vi "BooleanGame.vi"() -> ()   [LabVIEW 2015]
panel:
  out "String":string
  in  "Select a Puzzle":u16(ring) items=["None", "Puzzle 1", "Puzzle 2", "Puzzle 3", "Puzzle 4", "Puzzle 5", "Impossible Challenge"]
  in  "reset":bool
  in  "stop":bool
  in  "33":bool
  in  "23":bool
  in  "13":bool
  in  "32":bool
  in  "22":bool
  in  "12":bool
  in  "31":bool
  in  "21":bool
  in  "11":bool
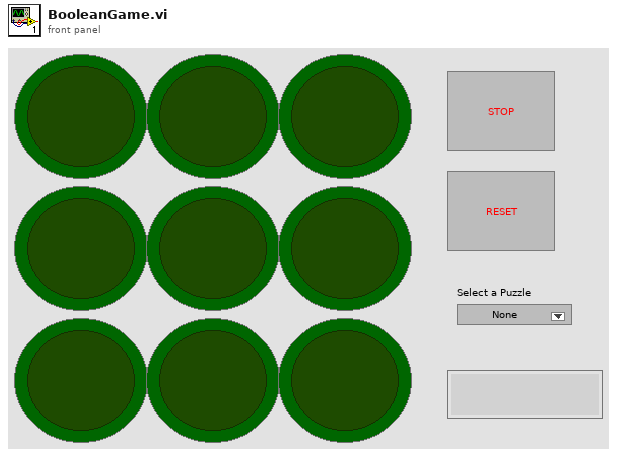
[diagram p1: front panel]
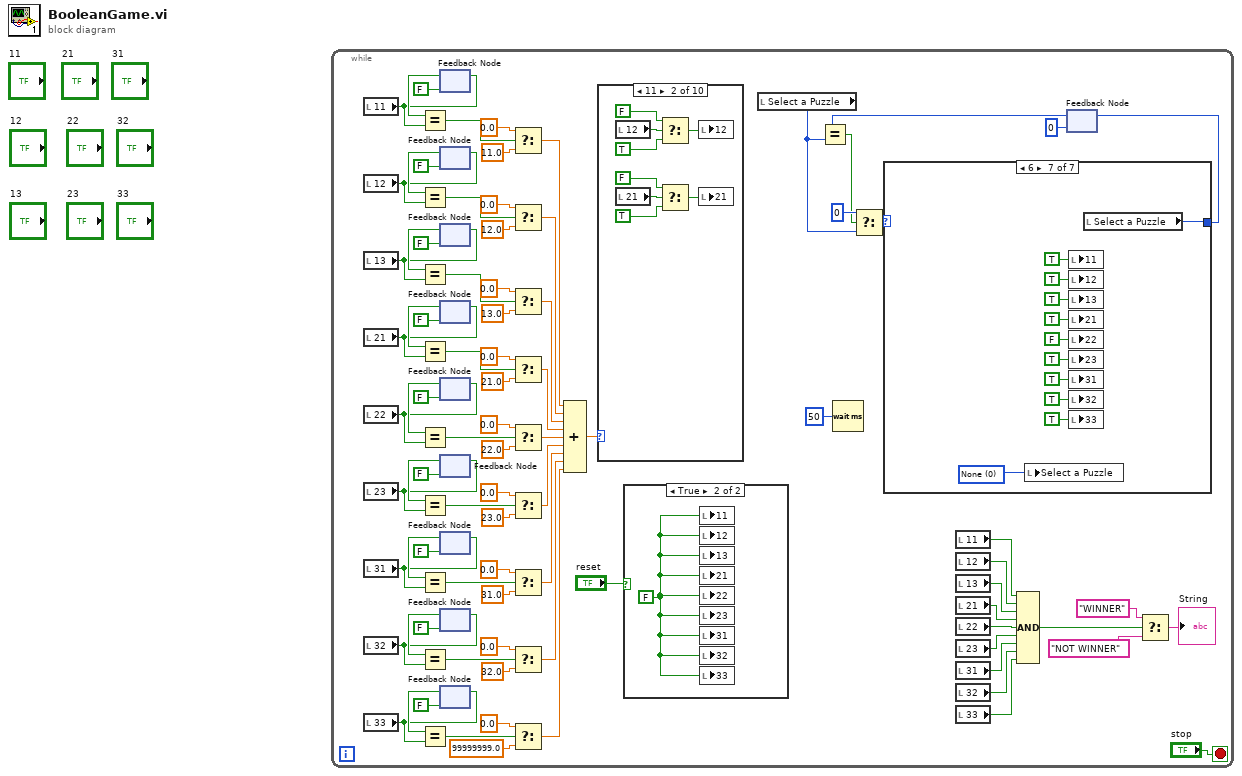
[diagram p0: block diagram]
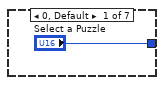
[diagram p2: hidden frame]
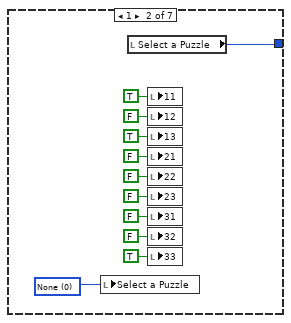
[diagram p3: hidden frame]
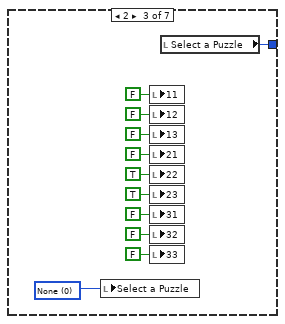
[diagram p4: hidden frame]
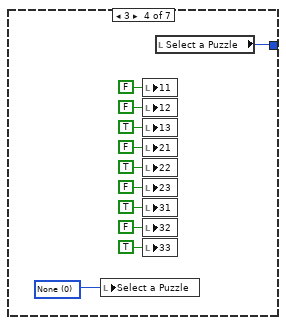
[diagram p5: hidden frame]
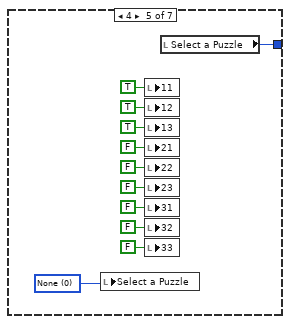
[diagram p6: hidden frame]
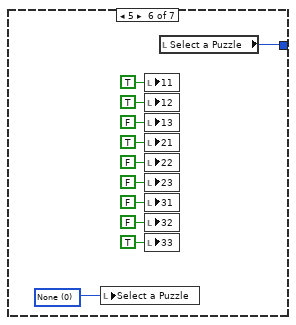
[diagram p7: hidden frame]
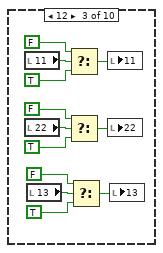
[diagram p10: hidden frame]
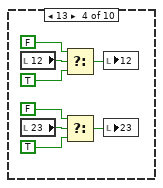
[diagram p11: hidden frame]
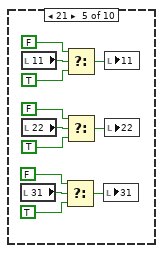
[diagram p12: hidden frame]
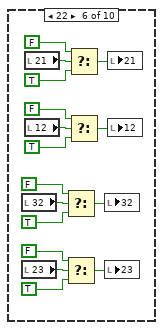
[diagram p13: hidden frame]
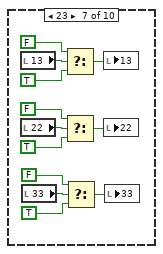
[diagram p14: hidden frame]
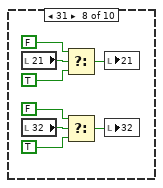
[diagram p15: hidden frame]
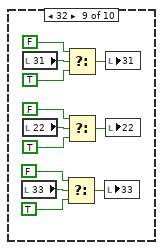
[diagram p16: hidden frame]
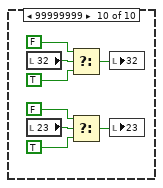
[diagram p17: hidden frame]
diagram:
  n1 = while {
    stop <- "stop" stop-if-true
    n2 = local read "11"() -> (w31:bool)
    n3 = local read "12"() -> (w30:bool)
    n4 = local read "13"() -> (w29:bool)
    n5 = local read "21"() -> (w28:bool)
    n6 = local read "22"() -> (w27:bool)
    n7 = local read "23"() -> (w26:bool)
    n8 = local read "31"() -> (w25:bool)
    n9 = local read "32"() -> (w24:bool)
    n10 = local read "33"() -> (w23:bool)
    n11 = feedback #1(FALSE) -> (w57:bool)
    n12 = Equal?(x=w57, y=w31) -> (x = y?=w58:bool)
    n13 = feedback-in #1(w31) -> ()
    n14 = feedback #2(FALSE) -> (w55:bool)
    n15 = Equal?(x=w55, y=w30) -> (x = y?=w56:bool)
    n16 = feedback-in #2(w30) -> ()
    n17 = feedback #3(FALSE) -> (w53:bool)
    n18 = Equal?(x=w53, y=w29) -> (x = y?=w54:bool)
    n19 = feedback-in #3(w29) -> ()
    n20 = feedback #4(FALSE) -> (w51:bool)
    n21 = Equal?(x=w51, y=w28) -> (x = y?=w52:bool)
    n22 = feedback-in #4(w28) -> ()
    n23 = feedback #5(FALSE) -> (w49:bool)
    n24 = Equal?(x=w49, y=w27) -> (x = y?=w50:bool)
    n25 = feedback-in #5(w27) -> ()
    n26 = feedback #6(FALSE) -> (w47:bool)
    n27 = Equal?(x=w47, y=w26) -> (x = y?=w48:bool)
    n28 = feedback-in #6(w26) -> ()
    n29 = feedback #7(FALSE) -> (w45:bool)
    n30 = Equal?(x=w45, y=w25) -> (x = y?=w46:bool)
    n31 = feedback-in #7(w25) -> ()
    n32 = feedback #8(FALSE) -> (w43:bool)
    n33 = Equal?(x=w43, y=w24) -> (x = y?=w44:bool)
    n34 = feedback-in #8(w24) -> ()
    n35 = feedback #9(FALSE) -> (w41:bool)
    n36 = Equal?(x=w41, y=w23) -> (x = y?=w42:bool)
    n37 = feedback-in #9(w23) -> ()
    n38 = Select(t=0.0, s=w58, f=11.0) -> (s? t:f=w68:dbl)
    n39 = Select(t=0.0, s=w56, f=12.0) -> (s? t:f=w67:dbl)
    n40 = Select(t=0.0, s=w54, f=13.0) -> (s? t:f=w66:dbl)
    n41 = Select(t=0.0, s=w52, f=21.0) -> (s? t:f=w65:dbl)
    n42 = Select(t=0.0, s=w50, f=22.0) -> (s? t:f=w64:dbl)
    n43 = Select(t=0.0, s=w48, f=23.0) -> (s? t:f=w63:dbl)
    n44 = Select(t=0.0, s=w46, f=31.0) -> (s? t:f=w62:dbl)
    n45 = Select(t=0.0, s=w44, f=32.0) -> (s? t:f=w61:dbl)
    n46 = Select(t=0.0, s=w42, f=99999999.0) -> (s? t:f=w60:dbl)
    n47 = Compound Arithmetic op=ADD(w68, w67, w66, w65, w64, w63, w62, w61, w60) -> (w59:dbl)
    n48 = case shown="11" w59 {
      frame 0, Default {
      }
      frame 11 {
        n49 = local read "12"() -> (w156:bool)
        n50 = local read "21"() -> (w163:bool)
        n51 = Select(t=FALSE, s=w156, f=TRUE) -> (s? t:f=w159:bool)
        n52 = Select(t=FALSE, s=w163, f=TRUE) -> (s? t:f=w160:bool)
        n53 = local write "12"(w159) -> ()
        n54 = local write "21"(w160) -> ()
      }
      frame 12 {
        n55 = local read "11"() -> (w168:bool)
        n56 = local read "22"() -> (w175:bool)
        n57 = local read "13"() -> (w164:bool)
        n58 = Select(t=FALSE, s=w168, f=TRUE) -> (s? t:f=w171:bool)
        n59 = Select(t=FALSE, s=w175, f=TRUE) -> (s? t:f=w172:bool)
        n60 = Select(t=FALSE, s=w164, f=TRUE) -> (s? t:f=w167:bool)
        n61 = local write "11"(w171) -> ()
        n62 = local write "22"(w172) -> ()
        n63 = local write "13"(w167) -> ()
      }
      frame 13 {
        n64 = local read "12"() -> (w176:bool)
        n65 = local read "23"() -> (w183:bool)
        n66 = Select(t=FALSE, s=w176, f=TRUE) -> (s? t:f=w179:bool)
        n67 = Select(t=FALSE, s=w183, f=TRUE) -> (s? t:f=w180:bool)
        n68 = local write "12"(w179) -> ()
        n69 = local write "23"(w180) -> ()
      }
      frame 21 {
        n70 = local read "31"() -> (w187:bool)
        n71 = local read "11"() -> (w188:bool)
        n72 = local read "22"() -> (w195:bool)
        n73 = Select(t=FALSE, s=w187, f=TRUE) -> (s? t:f=w184:bool)
        n74 = Select(t=FALSE, s=w188, f=TRUE) -> (s? t:f=w191:bool)
        n75 = Select(t=FALSE, s=w195, f=TRUE) -> (s? t:f=w192:bool)
        n76 = local write "31"(w184) -> ()
        n77 = local write "11"(w191) -> ()
        n78 = local write "22"(w192) -> ()
      }
      frame 22 {
        n79 = local read "32"() -> (w196:bool)
        n80 = local read "23"() -> (w203:bool)
        n81 = local read "21"() -> (w204:bool)
        n82 = local read "12"() -> (w211:bool)
        n83 = Select(t=FALSE, s=w196, f=TRUE) -> (s? t:f=w199:bool)
        n84 = Select(t=FALSE, s=w203, f=TRUE) -> (s? t:f=w200:bool)
        n85 = Select(t=FALSE, s=w204, f=TRUE) -> (s? t:f=w207:bool)
        n86 = Select(t=FALSE, s=w211, f=TRUE) -> (s? t:f=w208:bool)
        n87 = local write "32"(w199) -> ()
        n88 = local write "23"(w200) -> ()
        n89 = local write "21"(w207) -> ()
        n90 = local write "12"(w208) -> ()
      }
      frame 23 {
        n91 = local read "13"() -> (w216:bool)
        n92 = local read "22"() -> (w223:bool)
        n93 = local read "33"() -> (w215:bool)
        n94 = Select(t=FALSE, s=w216, f=TRUE) -> (s? t:f=w219:bool)
        n95 = Select(t=FALSE, s=w223, f=TRUE) -> (s? t:f=w220:bool)
        n96 = Select(t=FALSE, s=w215, f=TRUE) -> (s? t:f=w212:bool)
        n97 = local write "13"(w219) -> ()
        n98 = local write "22"(w220) -> ()
        n99 = local write "33"(w212) -> ()
      }
      frame 31 {
        n100 = local read "21"() -> (w224:bool)
        n101 = local read "32"() -> (w231:bool)
        n102 = Select(t=FALSE, s=w224, f=TRUE) -> (s? t:f=w227:bool)
        n103 = Select(t=FALSE, s=w231, f=TRUE) -> (s? t:f=w228:bool)
        n104 = local write "21"(w227) -> ()
        n105 = local write "32"(w228) -> ()
      }
      frame 32 {
        n106 = local read "33"() -> (w235:bool)
        n107 = local read "31"() -> (w236:bool)
        n108 = local read "22"() -> (w243:bool)
        n109 = Select(t=FALSE, s=w235, f=TRUE) -> (s? t:f=w232:bool)
        n110 = Select(t=FALSE, s=w236, f=TRUE) -> (s? t:f=w239:bool)
        n111 = Select(t=FALSE, s=w243, f=TRUE) -> (s? t:f=w240:bool)
        n112 = local write "33"(w232) -> ()
        n113 = local write "31"(w239) -> ()
        n114 = local write "22"(w240) -> ()
      }
      frame 99999999 {
        n115 = local read "32"() -> (w244:bool)
        n116 = local read "23"() -> (w251:bool)
        n117 = Select(t=FALSE, s=w244, f=TRUE) -> (s? t:f=w247:bool)
        n118 = Select(t=FALSE, s=w251, f=TRUE) -> (s? t:f=w248:bool)
        n119 = local write "32"(w247) -> ()
        n120 = local write "23"(w248) -> ()
      }
    }
    n121 = case shown="True" "reset" {
      frame False {
      }
      frame True {
        w155 = FALSE
        n122 = local write "11"(w155) -> ()
        n123 = local write "12"(w155) -> ()
        n124 = local write "13"(w155) -> ()
        n125 = local write "21"(w155) -> ()
        n126 = local write "22"(w155) -> ()
        n127 = local write "23"(w155) -> ()
        n128 = local write "31"(w155) -> ()
        n129 = local write "32"(w155) -> ()
        n130 = local write "33"(w155) -> ()
      }
    }
    n131 = local read "Select a Puzzle"() -> (w15:u16)
    n132 = Wait (ms)(milliseconds to wait=u32 50) -> ()  [unwired: 1 out]
    n133 = local read "11"() -> (w14:bool)
    n134 = local read "12"() -> (w13:bool)
    n135 = local read "13"() -> (w12:bool)
    n136 = local read "21"() -> (w11:bool)
    n137 = local read "22"() -> (w10:bool)
    n138 = local read "23"() -> (w9:bool)
    n139 = local read "31"() -> (w8:bool)
    n140 = local read "32"() -> (w7:bool)
    n141 = local read "33"() -> (w6:bool)
    n142 = Compound Arithmetic op=AND(w14, w13, w12, w11, w10, w9, w8, w7, w6) -> (w5:bool)
    n143 = feedback #10(u16 0 ("Select a Puzzle")) -> (w19:u16)
    n144 = Equal?(x=w19, y=w15) -> (x = y?=w16:bool)
    n145 = Select(t=u16 0 ("Select a Puzzle"), s=w16, f=w15) -> (s? t:f=w18:u16)
    n146 = case shown="6" w18 {
      tunnel: ["Select a Puzzle" w99 w110 w121 w132 w143 w154] -> w21
      frame 0, Default {
      }
      frame 1 {
        w89 = u16 0 items=["None", "Puzzle 1", "Puzzle 2", "Puzzle 3", "Puzzle 4", "Puzzle 5"] ("Select a Puzzle")
        n147 = local write "Select a Puzzle"(w89) -> ()
        n148 = local read "Select a Puzzle"() -> (w99:u16)
        n149 = local write "11"(TRUE ("11")) -> ()
        n150 = local write "12"(FALSE ("12")) -> ()
        n151 = local write "13"(TRUE ("13")) -> ()
        n152 = local write "21"(FALSE ("21")) -> ()
        n153 = local write "22"(FALSE ("22")) -> ()
        n154 = local write "23"(FALSE ("23")) -> ()
        n155 = local write "31"(FALSE ("31")) -> ()
        n156 = local write "32"(FALSE ("32")) -> ()
        n157 = local write "33"(TRUE ("33")) -> ()
      }
      frame 2 {
        w100 = u16 0 items=["None", "Puzzle 1", "Puzzle 2", "Puzzle 3", "Puzzle 4", "Puzzle 5"] ("Select a Puzzle")
        n158 = local write "Select a Puzzle"(w100) -> ()
        n159 = local write "11"(FALSE ("11")) -> ()
        n160 = local write "12"(FALSE ("12")) -> ()
        n161 = local write "13"(FALSE ("13")) -> ()
        n162 = local write "21"(FALSE ("21")) -> ()
        n163 = local write "22"(TRUE ("22")) -> ()
        n164 = local write "23"(TRUE ("23")) -> ()
        n165 = local write "31"(FALSE ("31")) -> ()
        n166 = local write "32"(FALSE ("32")) -> ()
        n167 = local write "33"(FALSE ("33")) -> ()
        n168 = local read "Select a Puzzle"() -> (w110:u16)
      }
      frame 3 {
        w111 = u16 0 items=["None", "Puzzle 1", "Puzzle 2", "Puzzle 3", "Puzzle 4", "Puzzle 5"] ("Select a Puzzle")
        n169 = local write "Select a Puzzle"(w111) -> ()
        n170 = local write "11"(FALSE ("11")) -> ()
        n171 = local write "12"(FALSE ("12")) -> ()
        n172 = local write "13"(TRUE ("13")) -> ()
        n173 = local write "21"(FALSE ("21")) -> ()
        n174 = local write "22"(TRUE ("22")) -> ()
        n175 = local write "23"(FALSE ("23")) -> ()
        n176 = local write "31"(TRUE ("31")) -> ()
        n177 = local write "32"(FALSE ("32")) -> ()
        n178 = local write "33"(TRUE ("33")) -> ()
        n179 = local read "Select a Puzzle"() -> (w121:u16)
      }
      frame 4 {
        w122 = u16 0 items=["None", "Puzzle 1", "Puzzle 2", "Puzzle 3", "Puzzle 4", "Puzzle 5"] ("Select a Puzzle")
        n180 = local write "Select a Puzzle"(w122) -> ()
        n181 = local write "11"(TRUE ("11")) -> ()
        n182 = local write "12"(TRUE ("12")) -> ()
        n183 = local write "13"(TRUE ("13")) -> ()
        n184 = local write "21"(FALSE ("21")) -> ()
        n185 = local write "22"(FALSE ("22")) -> ()
        n186 = local write "23"(FALSE ("23")) -> ()
        n187 = local write "31"(FALSE ("31")) -> ()
        n188 = local write "32"(FALSE ("32")) -> ()
        n189 = local write "33"(FALSE ("33")) -> ()
        n190 = local read "Select a Puzzle"() -> (w132:u16)
      }
      frame 5 {
        w133 = u16 0 items=["None", "Puzzle 1", "Puzzle 2", "Puzzle 3", "Puzzle 4", "Puzzle 5"] ("Select a Puzzle")
        n191 = local write "Select a Puzzle"(w133) -> ()
        n192 = local write "11"(TRUE ("11")) -> ()
        n193 = local write "12"(TRUE ("12")) -> ()
        n194 = local write "13"(FALSE ("13")) -> ()
        n195 = local write "21"(TRUE ("21")) -> ()
        n196 = local write "22"(FALSE ("22")) -> ()
        n197 = local write "23"(FALSE ("23")) -> ()
        n198 = local write "31"(FALSE ("31")) -> ()
        n199 = local write "32"(FALSE ("32")) -> ()
        n200 = local write "33"(TRUE ("33")) -> ()
        n201 = local read "Select a Puzzle"() -> (w143:u16)
      }
      frame 6 {
        w144 = u16 0 items=["None", "Puzzle 1", "Puzzle 2", "Puzzle 3", "Puzzle 4", "Puzzle 5"] ("Select a Puzzle")
        n202 = local write "Select a Puzzle"(w144) -> ()
        n203 = local write "11"(TRUE ("11")) -> ()
        n204 = local write "12"(TRUE ("12")) -> ()
        n205 = local write "13"(TRUE ("13")) -> ()
        n206 = local write "21"(TRUE ("21")) -> ()
        n207 = local write "22"(FALSE ("22")) -> ()
        n208 = local write "23"(TRUE ("23")) -> ()
        n209 = local write "31"(TRUE ("31")) -> ()
        n210 = local write "32"(TRUE ("32")) -> ()
        n211 = local write "33"(TRUE ("33")) -> ()
        n212 = local read "Select a Puzzle"() -> (w154:u16)
      }
    }
    n213 = feedback-in #10(w21) -> ()
    n214 = Select(t="WINNER", s=w5, f="NOT WINNER") -> (s? t:f=→"String":string)
  }
